vi "TCam_Overlay_Fixedpoint.vi"(8 "error in (no error)":errorcluster, 9 "Line Width":u32=1 min=1, 10 "Line Length":u16=1 min=1, 11 "output cluster":T2={"Core"={"Current VI Reference"=refnum, "Close Panel on Exit?"=FALSE}, "Image Out"="img_in", "State"=1, "Points"={"Top Left"={"X"=0.0, "Y"=0.0}, "Top Right"={"X"=0.0, "Y"=0.0}, "Bottom Left"={"X"=0.0, "Y"=0.0}, "Bottom Right"={"X"=0.0, "Y"=0.0}, "x space 2"=0.0, "y space 2"=0.0, "x_space"=0.0, "y_space"=0.0, "Pixels"=[], "Fixpoint"={"X"=539.0, "Y"=75.0}}, "img_array"=[], "Temps"=[], "Temps_Array"=[]} {"Points"."Top Left"."Y" format="%.2f"; "Points"."Top Left"."X" format="%.2f"; "Points"."Top Right"."Y" format="%.2f"; "Points"."Top Right"."X" format="%.2f"; "Points"."Bottom Left"."Y" format="%.2f"; "Points"."Bottom Left"."X" format="%.2f"; "Points"."Bottom Right"."Y" format="%.2f"; "Points"."Bottom Right"."X" format="%.2f"; "Points"."Fixpoint"."Y" format="%.2f"; "Points"."Fixpoint"."X" format="%.2f"}) -> (0 "error out":errorcluster={"status"=TRUE, "code"=-1074396120, "source"="IMAQ Overlay Lines\n  "}, 3 "Image Out":T1)   [LabVIEW 2020]
uses:
  DataCluster_TCAL.ctl
  <vilib>/vision/Image Controls.llb/IMAQ Image.ctl
panel:
  out "Array":cluster{"X":dbl, "Y":dbl}[](array[cluster])=[{"X"=539.0, "Y"=76.0}, {"X"=539.0, "Y"=74.0}, {"X"=538.0, "Y"=75.0}, {"X"=540.0, "Y"=75.0}]
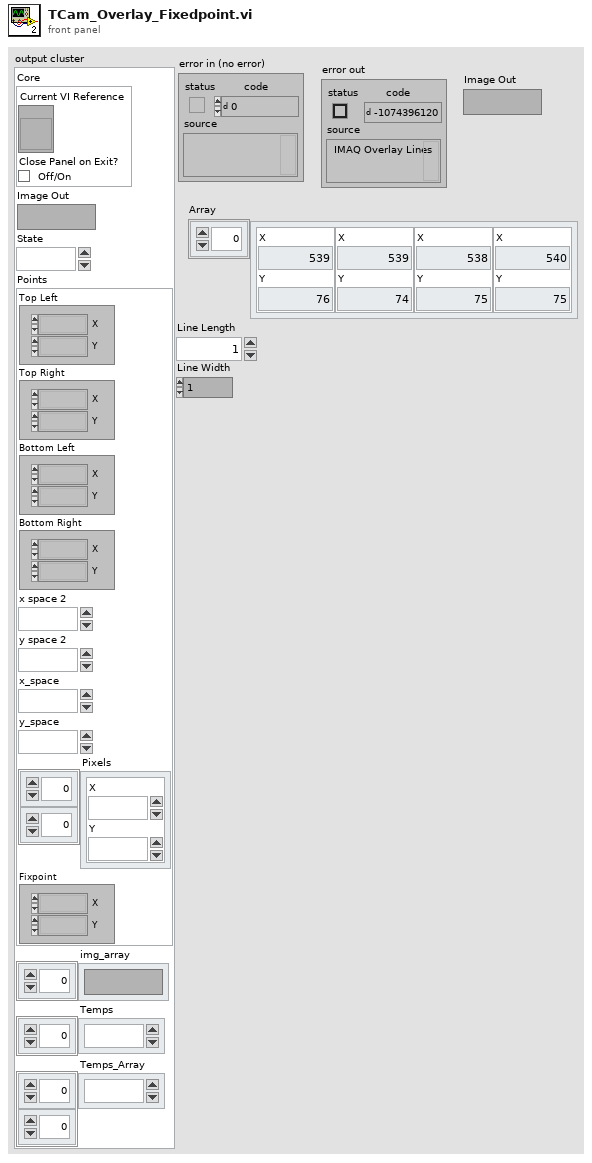
[diagram p1: front panel]
types:
  T1 = typedef "IMAQ Image.ctl" = refnum<image>
  T2 = typedef "DataCluster_TCAL.ctl" = cluster{"Core":cluster{"Current VI Reference":refnum<vi>, "Close Panel on Exit?":bool}, "Image Out":T1, "State":i32, "Points":cluster{"Top Left":T3, "Top Right":T3, "Bottom Left":T3, "Bottom Right":T3, "x space 2":dbl, "y space 2":sgl, "x_space":sgl, "y_space":sgl, "Pixels":cluster{"X":i32, "Y":i32}[][], "Fixpoint":T3}, "img_array":T1[], "Temps":dbl[], "Temps_Array":dbl[][]}
  T3 = typedef "IMAQ Point" = cluster{"X":sgl, "Y":sgl}
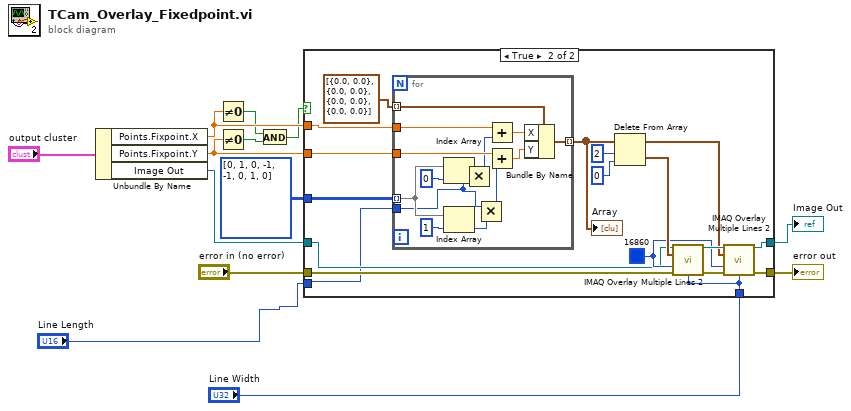
[diagram p0: block diagram]
diagram:
  n1 = Unbundle By Name("output cluster") -> ("Points.Fixpoint.X"=w13:sgl, "Points.Fixpoint.Y"=w12:sgl, "Image Out"=w4:T1)
  n2 = Not Equal To 0?(x=w13) -> (x != 0?=w8:bool)
  n3 = Not Equal To 0?(x=w12) -> (x != 0?=w9:bool)
  n4 = And(x=w8, y=w9) -> (x .and. y?=w10:bool)
  n5 = case shown="True" w10 {
    tunnel: i32[][] [[0, 1], [0, -1], [-1, 0], [1, 0]] -> [_ w33]
    tunnel: w12 -> [_ w32]
    tunnel: w13 -> [_ w31]
    tunnel: w4 -> [w14 w21]
    tunnel: "error in (no error)" -> [w15 w20]
    tunnel: [w15 w19] -> w5
    tunnel: [w14 w18] -> w3
    tunnel: "Line Length" -> [_ w17]
    tunnel: "Line Width" -> [_ w16]
    frame False {
    }
    frame True {
      w23 = u32 16860 ("Color")
      n6 = for {
        tunnel: w33 -> [w46] mode=indexing
        tunnel: w32 -> [w42]
        tunnel: w31 -> [w44]
        tunnel: cluster{"X":dbl, "Y":dbl}[] [{"X"=0.0, "Y"=0.0}, {"X"=0.0, "Y"=0.0}, {"X"=0.0, "Y"=0.0}, {"X"=0.0, "Y"=0.0}] ("Line End Points") -> [w40] mode=indexing
        tunnel: [w37] -> w27 mode=indexing
        tunnel: w17 -> [w34]
        n7 = Index Array(array=w46, index=0) -> (element=w43:i32)
        n8 = Index Array(array=w46, index=1) -> (element=w41:i32)
        n9 = Multiply(x=w34, y=w43) -> (x*y=w36:i32)
        n10 = Multiply(x=w34, y=w41) -> (x*y=w35:i32)
        n11 = Add(x=w44, y=w36) -> (x+y=w39:sgl)
        n12 = Add(x=w42, y=w35) -> (x+y=w38:sgl)
        n13 = Bundle By Name(cluster=w40, "X"=w39, "Y"=w38) -> (w37:cluster{"X":dbl, "Y":dbl})
      }
      "Array" <- w27
      n14 = Delete From Array(array=w27, length=2 ("index"), index=0 ("length")) -> (deleted portion=w26:cluster{"X":dbl, "Y":dbl}[], array with subset deleted=w24:cluster{"X":dbl, "Y":dbl}[])
      n15 = call "IMAQ Overlay Multiple Lines 2"("Image"=w21, "Line End Points"=w26, "Color"=w23, "error in (no error)"=w20, "Width"=w16) -> ("Image Out"=w25:T1, "error out"=w22:errorcluster)  [unwired: 9 in]
      n16 = call "IMAQ Overlay Multiple Lines 2"("Image"=w25, "Line End Points"=w24, "Color"=w23, "error in (no error)"=w22, "Width"=w16) -> ("Image Out"=w18:T1, "error out"=w19:errorcluster)  [unwired: 9 in]
    }
  }
  "error out" <- w5
  "Image Out" <- w3
